vi "TCL Select Base Fragments NfragsNcriteria.vi"(3 "error in (no error)":errorcluster, 4 "criteria":T1(array[cluster]), 5 "fragments":string[](array[string])) -> (0 "error out":errorcluster, 1 "matches":string[][](array[string]), 2 "fragments out":string[](array[string]))   [LabVIEW 2010]
uses:
  TCL Global.vi
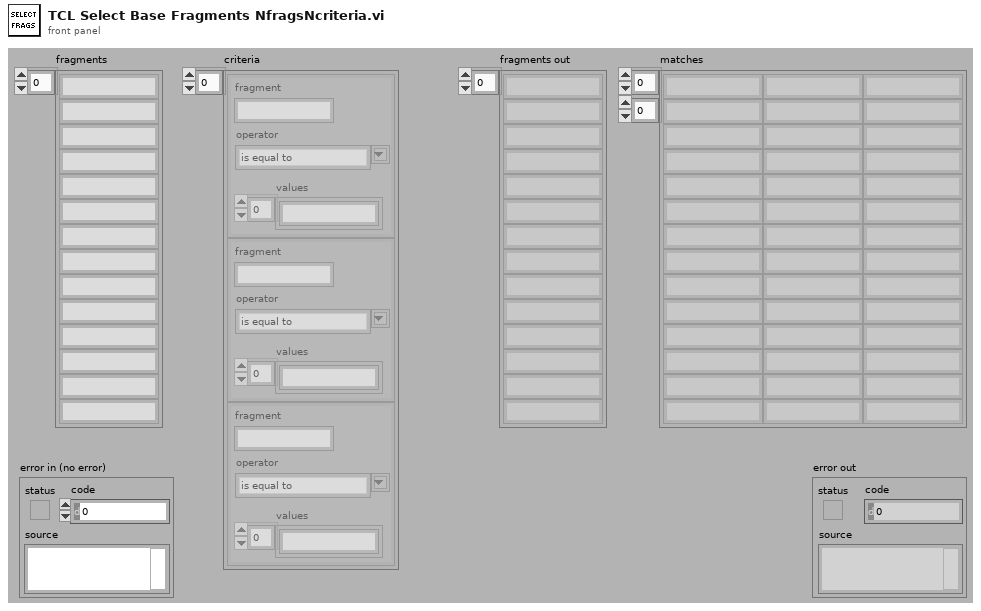
[diagram p1: front panel]
types:
  T1 = cluster{"fragment":string, "values":string[], "operator":string}[]
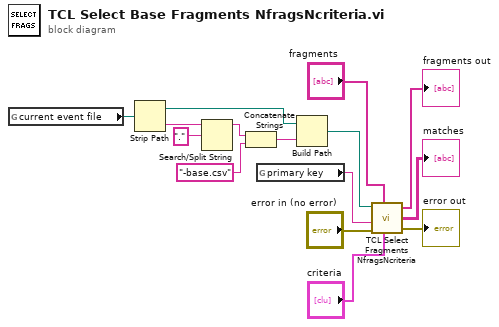
[diagram p0: block diagram]
diagram:
  n1 = global read "TCL Global.vi" "current event file"() -> (w7:path)
  n2 = Strip Path(path=w7) -> (stripped path=w6:path, name=w5:string)
  n3 = Search/Split String(string=w5, search string/char (-)=".") -> (substring before match=w1:string)  [unwired: 1 in, 2 out]
  n4 = Concatenate Strings(w1, "-base.csv" ("string")) -> (w3:string)
  n5 = global read "TCL Global.vi" "primary key"() -> (w9:string)
  n6 = Build Path(base path=w6, name or relative path=w3) -> (appended path=w2:path)
  n7 = call "TCL Select Fragments NfragsNcriteria.vi"("event file"=w2, "fragments"="fragments", "primary key"=w9, "criteria"="criteria", "error in (no error)"="error in (no error)") -> ("fragments out"=→"fragments out":string[], "matches"=→"matches":string[][], "error out"=→"error out":errorcluster)  [unwired: 1 in]
